vi "Rotate24bit.vi"(1 "image data":T1, 2 "theta (deg)":dbl(slide) scale=-180.0..180.0) -> (0 "image data 2":T1)   [LabVIEW 2017]
uses:
  <vilib>/picture/picture.llb/imagedata.ctl
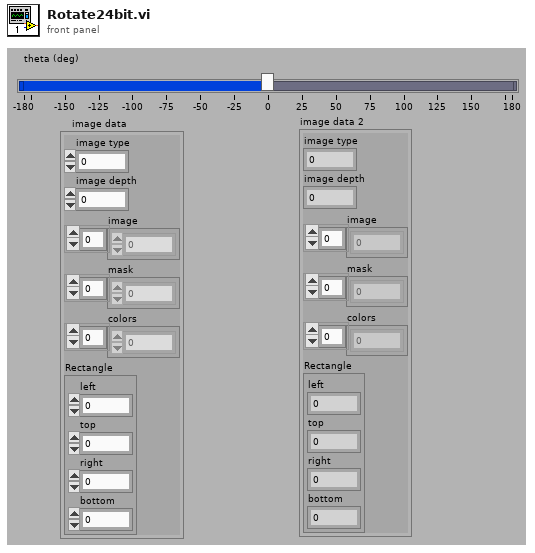
[diagram p1: front panel]
types:
  T1 = typedef "imagedata.ctl" = cluster{"image type":i32, "image depth":i32, "image":u8[], "mask":u8[], "colors":u32[], "Rectangle":cluster{"left":i16, "top":i16, "right":i16, "bottom":i16}}
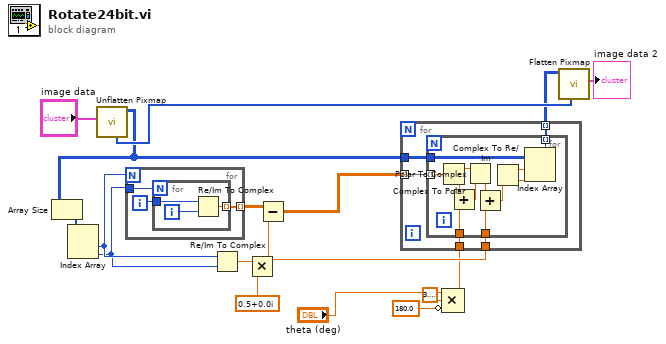
[diagram p0: block diagram]
diagram:
  n1 = call <vilib>:"Unflatten Pixmap.vi"("image data"="image data") -> ("24-bit pixmap"=w2:u32[][], "colors"=w9:u32[])  [unwired: 4 in, 5 out]
  n2 = Array Size(array=w2) -> (size(s)=w14:i32[])
  n3 = Index Array(array=w14) -> (element #1=w13:i32, element #2=w12:i32)  [unwired: 2 in]
  n4 = for {
    N: w13 -> [_]
    tunnel: w12 -> [w20]
    tunnel: [w18] -> w17 mode=indexing
    i -> [w19]
    n5 = for {
      N: w20 -> [_]
      tunnel: w19 -> [w22]
      tunnel: [w21] -> w18 mode=indexing
      i -> [w23]
      n6 = Re/Im To Complex(1:w23, 2:w22) -> (0:w21:cdb)
    }
  }
  n7 = Re/Im To Complex(1:w12, 2:w13) -> (0:w15:cdb)
  n8 = Multiply(x=w15, y=cdb 0.5+0.0i) -> (x*y=w11:cdb)
  n9 = Subtract(x=w17, y=w11) -> (x-y=w16:cdb[][])
  n10 = Compound Arithmetic op=MULTIPLY("theta (deg)", 3.141592653589793, invert 180.0 ("value")) -> (w5:dbl)
  n11 = for {
    tunnel: w5 -> [w28]
    tunnel: w2 -> [w27]
    tunnel: w11 -> [w26]
    tunnel: w16 -> [w25] mode=indexing
    tunnel: [w24] -> w1 mode=indexing
    n12 = for {
      tunnel: w27 -> [w34]
      tunnel: w28 -> [w37]
      tunnel: w26 -> [w31]
      tunnel: w25 -> [w30] mode=indexing
      tunnel: [w29] -> w24 mode=indexing
      n13 = Complex To Polar(r * e^(i*theta)=w30) -> (r=w40:dbl, theta=w39:dbl)
      n14 = Add(x=w39, y=w37) -> (x+y=w38:dbl)
      n15 = Polar To Complex(1:w38, 2:w40) -> (0:w36:cdb)
      n16 = Add(x=w36, y=w31) -> (x+y=w32:cdb)
      n17 = Complex To Re/Im(x + iy=w32) -> (x=w35:dbl, y=w33:dbl)
      n18 = Index Array(array=w34, index (row)=w35, index (col)=w33) -> (element=w29:u32)
    }
  }
  n19 = call <vilib>:"Flatten Pixmap.vi"("colors"=w9, "24-bit pixmap"=w1) -> ("image data"=→"image data 2":T1)  [unwired: 9 in]
